vi "PRIME Detector Check Files and Add FITS data.vi"(5 "Observation":T2={"Priority"=0, "ID"="", "Observer"="", "Obj Name"="", "Obj Type"="", "RA and DEC String"={"RA"="HH:MM:SS.nnn", "DEC"="DEG:arcmin:arcsec.nn"}, "Filter Wheel 1"="", "Filter Wheel 2"="", "Integration Time"=0.0, "Observation Status"=enum."Error", "Offsets"={"RA"=0.0, "DEC"=0.0, "ROT"=0.0}, "Images"=0, "Dither Options"={"Dither"=enum."None", "Dither Radius"=0.0, "Dither Points"=0, "Dither Phase"=0.0}, "Comment 1"="", "Comment 2"=""}, 7 "Detector Config":T7={"Detector"=0, "Offsets"=[[0, 0, 0, 0, 0, 0, 0, 0, 0, 0, 0, 0, 0, 0, 0, 0, 0, 0, 0, 0, 0, 0, 0, 0, 0, 0, 0, 0, 0, 0, 0, 0]], "Detector Computer"={"Machine"="192.168.121.11", "Password"="rSL!nux23456", "FITS File Path"="", "Port"=44444, "Header Path"="", "Name"=""}, "FITS hdr template0"=path "", "FITS hdr template1"=path "", "FITS Data File Path"=path "", "FITS Detector Settings"={"Exp Time Short"=0.0, "# of Frames"=0.0, "Exp Time Long"=0.0, "# of Groups"=0.0, "Object Name"="", "Object"="", "Obs Type"="", "Image Type"="", "Observer"="", "Observer Affiliation"=""}, "Sim Folder"=path "", "Integration Mode"=enum."SSR", "Integration Time"=0.0, "Frame Int Time"=0.0} {"Offsets" format="%04x"; "Detector" items=["0", "1", "2"]}, 8 "error in (no error)":errorcluster, 10 "Image Array":cluster{"CAMERA3":string[]}[](array[cluster]), 11 "Map in":map{string, T1}(c390)) -> (0 "error out":errorcluster, 3 "Map out":map{string, T1}(c390))   [LabVIEW 2024]
uses:
  RIMAS Detector Config.ctl
  RIMAS Detector Server Config.ctl
  RIMAS Observation Config.ctl
  Detector enum Detector Integration Mode.ctl
  typedefs/CC cluster Observation.ctl
  Observation Queue/CC enum Observation Status.ctl
  Telescope/CC cluster Telescope Offsets.ctl
  typedefs/CC cluster Observation Dither Options.ctl
  typedefs/CC enum Dither Selection.ctl
  Detector Image typedef cluster.ctl
  Detector Class.lvclass
panel:
  # "sec"
  # "sec"
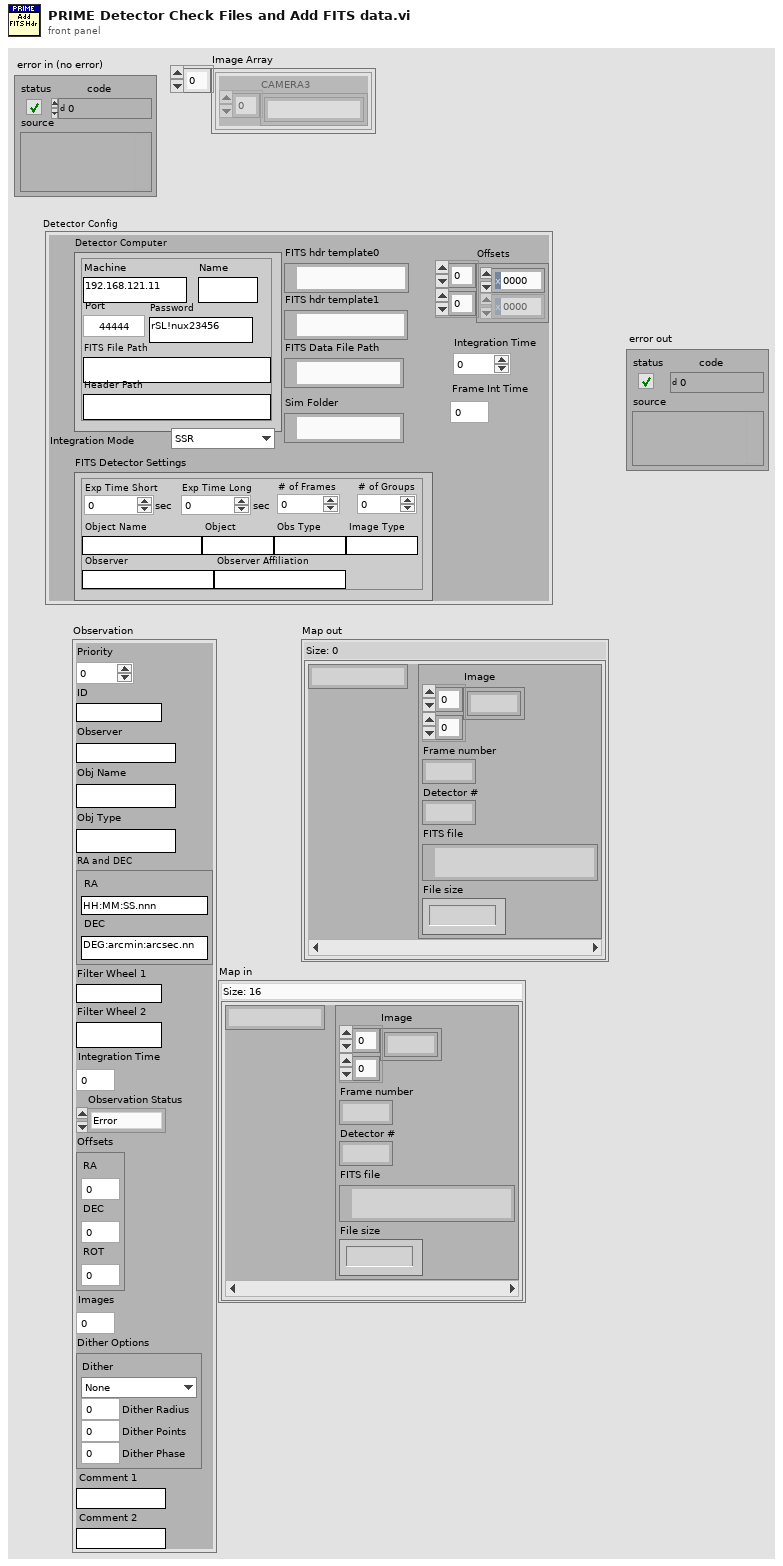
[diagram p1: front panel]
types:
  T1 = typedef "Detector Class.lvclass/Detector Image typedef cluster.ctl" = cluster{"Image":sgl[][], "Frame number":i32, "Detector #":u16, "FITS file":path, "File size":i64}
  T2 = typedef "CC cluster Observation.ctl" = cluster{"Priority":i32, "ID":string, "Observer":string, "Obj Name":string, "Obj Type":string, "RA and DEC String":cluster{"RA":string, "DEC":string}, "Filter Wheel 1":string, "Filter Wheel 2":string, "Integration Time":dbl, "Observation Status":T3, "Offsets":T4, "Images":i32, "Dither Options":T5, "Comment 1":string, "Comment 2":string}
  T3 = typedef "CC enum Observation Status.ctl" = enum16{"Ready", "Running", "Done", "Error"}
  T4 = typedef "CC cluster Telescope Offsets.ctl" = cluster{"RA":dbl, "DEC":dbl, "ROT":dbl}
  T5 = typedef "CC cluster Observation Dither Options.ctl" = cluster{"Dither":T6, "Dither Radius":dbl, "Dither Points":i32, "Dither Phase":dbl}
  T6 = typedef "CC enum Dither Selection.ctl" = enum16{"None", "Circle", "Random"}
  T7 = typedef "RIMAS Detector Config.ctl" = cluster{"Detector":u16, "Offsets":u16[][], "Detector Computer":T8, "FITS hdr template0":path, "FITS hdr template1":path, "FITS Data File Path":path, "FITS Detector Settings":T9, "Sim Folder":path, "Integration Mode":T10, "Integration Time":dbl, "Frame Int Time":dbl}
  T8 = typedef "RIMAS Detector Server Config.ctl" = cluster{"Machine":string, "Password":string, "FITS File Path":string, "Port":u16, "Header Path":string, "Name":string}
  T9 = typedef "RIMAS Observation Config.ctl" = cluster{"Exp Time Short":dbl, "# of Frames":dbl, "Exp Time Long":dbl, "# of Groups":dbl, "Object Name":string, "Object":string, "Obs Type":string, "Image Type":string, "Observer":string, "Observer Affiliation":string}
  T10 = typedef "Detector enum Detector Integration Mode.ctl" = enum16{"SSR", "CDS", "MEAN", "MEDIAN", "MODE", "MIIN", "MAX"}
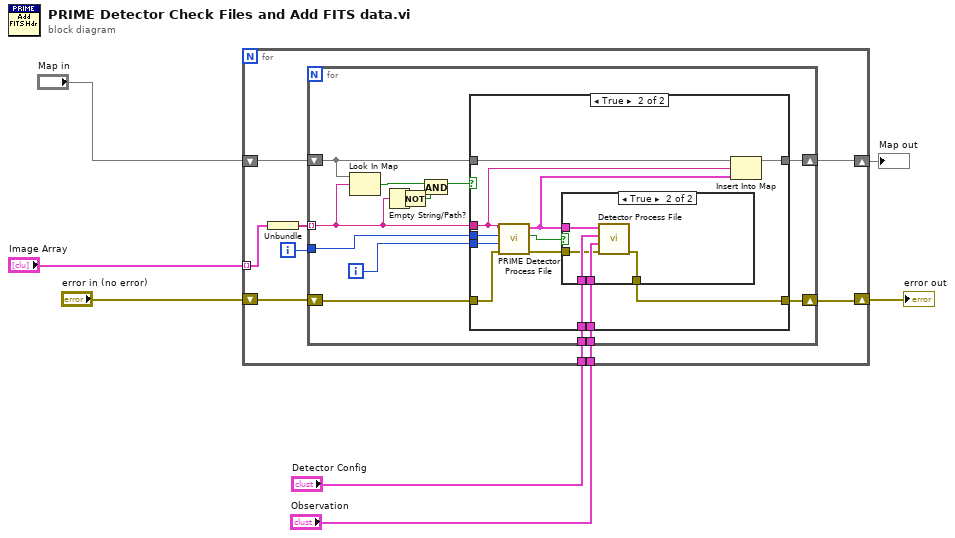
[diagram p0: block diagram]
diagram:
  n1 = for {
    shift-right: [w12] -> w3
    shift-left: "Map in" -> [w16]
    tunnel: "Image Array" -> [w15] mode=indexing
    tunnel: "Detector Config" -> [w11]
    tunnel: "Observation" -> [w10]
    shift-right: [w8] -> w1
    shift-left: "error in (no error)" -> [w9]
    i -> [w13]
    n2 = Unbundle(w15) -> ("CAMERA3"=w14:string[])
    n3 = for {
      shift-right: [w25] -> w12
      shift-left: w16 -> [w26]
      tunnel: w14 -> [w20] mode=indexing
      tunnel: w13 -> [w28]
      tunnel: w11 -> [w24]
      tunnel: w10 -> [w23]
      shift-right: [w21] -> w8
      shift-left: w9 -> [w22]
      i -> [w27]
      n4 = Look In Map(map=w26, key=w20) -> (key not found?=w29:bool)  [unwired: 1 in, 1 out]
      n5 = Empty String/Path?(string/path=w20) -> (empty?=w18:bool)
      n6 = Not(x=w18) -> (.not. x?=w17:bool)
      n7 = And(x=w29, y=w17) -> (x .and. y?=w19:bool)
      n8 = case shown="True" w19 {
        tunnel: w20 -> [_ w40]
        tunnel: w28 -> [_ w43]
        tunnel: w27 -> [_ w42]
        tunnel: w26 -> [w31 w41]
        tunnel: [w31 w38] -> w25
        tunnel: w24 -> [_ w37]
        tunnel: w23 -> [_ w36]
        tunnel: w22 -> [w30 w35]
        tunnel: [w30 w33] -> w21
        frame False {
        }
        frame True {
          n9 = call "PRIME Detector Process File.vi"("error in (no error)"=w35, "Frame"=w42, "Camera"=w43, "Filename"=w40) -> ("error out"=w34:errorcluster, "Keep?"=w32:bool, "Image Data"=w39:T1)  [unwired: 5 in]
          n10 = case shown="True" w32 {
            tunnel: w39 -> [_ w49]
            tunnel: w37 -> [_ w48]
            tunnel: w36 -> [_ w47]
            tunnel: w34 -> [w44 w46]
            tunnel: [w44 w45] -> w33
            frame False {
            }
            frame True {
              n11 = call "Detector Process File.vi"("error in (no error)"=w46, "Observation"=w47, "Detector Config"=w48, "Image"=w49) -> ("error out"=w45:errorcluster)  [unwired: 6 in, 1 out]
            }
          }
          n12 = Insert Into Map(map in=w41, key=w40, value=w39) -> (map out=w38:map{string, T1})  [unwired: 2 out]
        }
      }
    }
  }
  "error out" <- w1
  "Map out" <- w3
